vi "Doc_Builder_Write_Horz_Line.vi"(11 "NI_report in":refnum<class "NI_report.lvclass">) -> (3 "NI_report out":refnum<class "NI_report.lvclass">)   [LabVIEW 2019]
uses:
  <vilib>/Utility/NIReport.llb/NI_report.lvclass
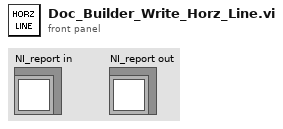
[diagram p1: front panel]
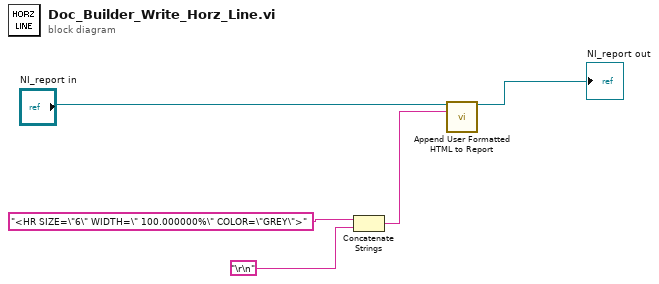
[diagram p0: block diagram]
diagram:
  n1 = Concatenate Strings("<HR SIZE=\"6\" WIDTH=\" 100.000000%\" COLOR=\"GREY\">" ("text"), "\r\n") -> (w1:string)
  n2 = call-dynamic "Append User Formatted HTML to Report.vi"("report in"="NI_report in", "HTML text"=w1) -> ("report out"=→"NI_report out":refnum<class "NI_report.lvclass">)  [unwired: 12 in, 1 out]
